vi "AB_Engine_Copy_Error_Files.vi"(8 "error in (no error)":errorcluster, 10 "preview only?":bool, 11 "Error destination path":path) -> (0 "error out":errorcluster, 3 "copied error files":path[](array[path]))   [LabVIEW 2020]
doc: "If \"Error destination path\" is empty, the computed RTE location is used."
uses:
  <resource>/Framework/Providers/Common/provcom_StringGlobals.vi
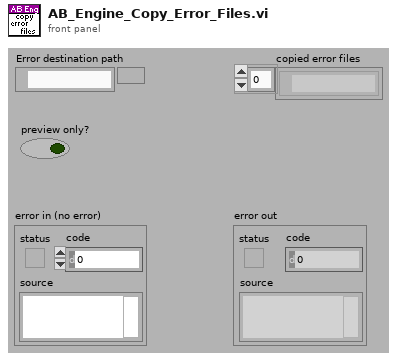
[diagram p1: front panel]
types:
  T1 = cluster{"base path":path, "relative path":path}[]
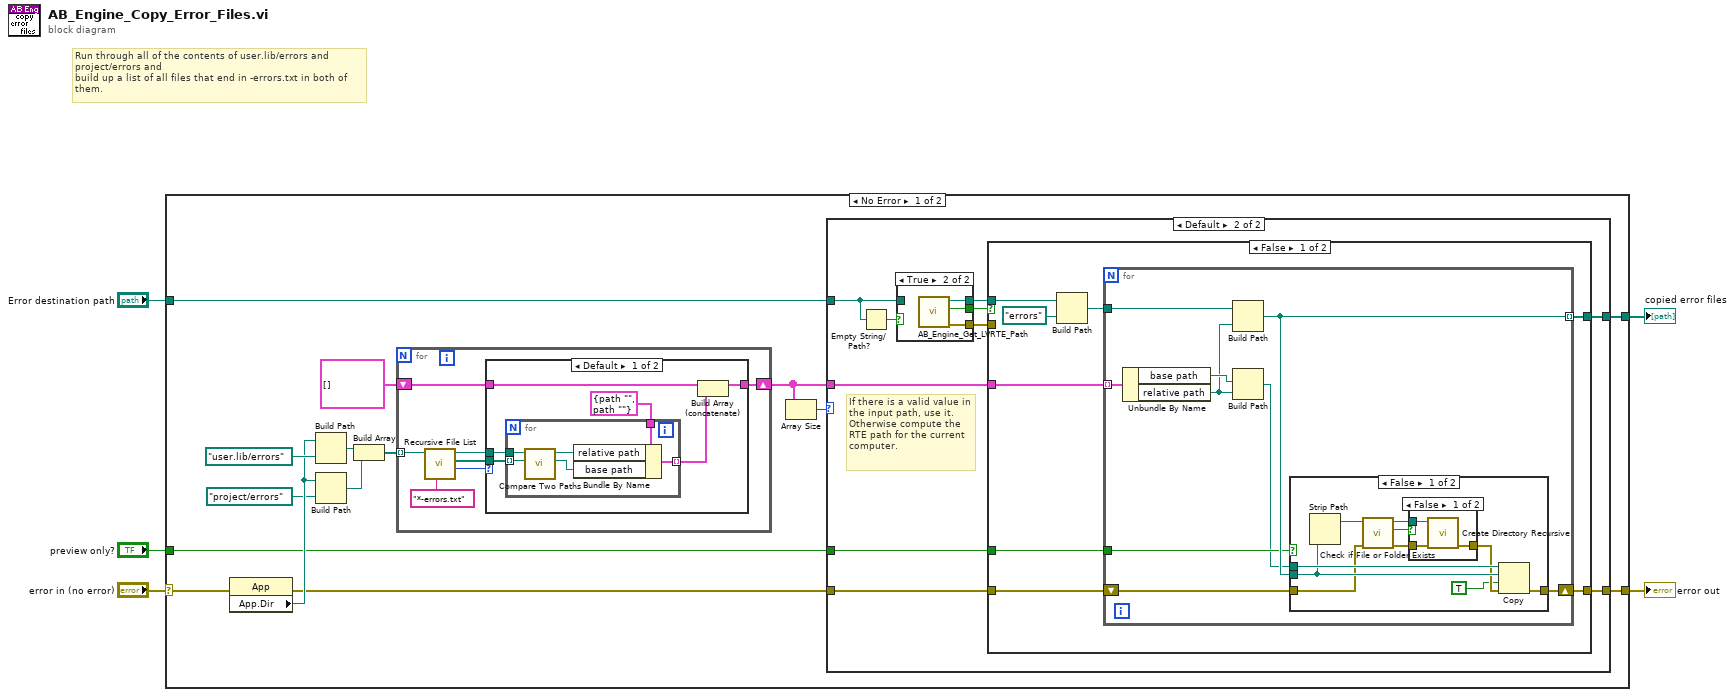
[diagram p0: block diagram]
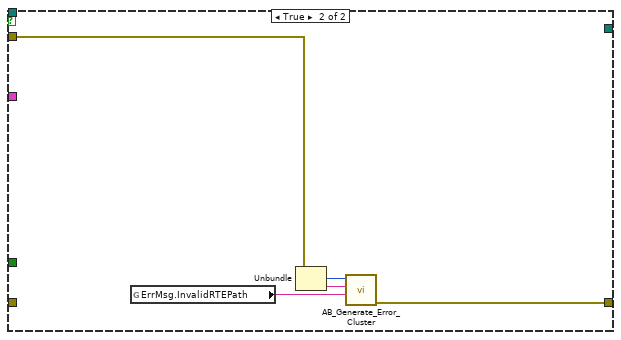
[diagram p5: hidden frame]
diagram:
  # "Run through all of the contents of user.lib/errors and project/errors and\nbuild up a list of all files that end in -errors.txt in both of them."
  n1 = case shown="No Error" "error in (no error)" {
    selector: "error in (no error)" -> [w19 w93]
    tunnel: [w20 w93] -> w4
    tunnel: "Error destination path" -> [w6 _]
    tunnel: [w11 _] -> w2
    tunnel: "preview only?" -> [w10 _]
    frame No Error {
      n2 = property class="App"(error in=w19) -> (error out=w9:errorcluster, "App.Dir"=w17:path)  [unwired: 1 in, 1 out]
      n3 = Build Path(base path=w17, name or relative path=path "user.lib/errors") -> (appended path=w15:path)
      n4 = Build Path(base path=w17, name or relative path=path "project/errors") -> (appended path=w14:path)
      n5 = Build Array(w15, w14) -> (w13:path[])
      n6 = for {
        shift-right: [w74] -> w8
        shift-left: T1 [] -> [w79]
        tunnel: w13 -> [w78] mode=indexing
        n7 = call <vilib>:"Recursive File List.vi"("pattern"="*-errors.txt" ("regular expression"), "Folder Path"=w78) -> ("Number of Files"=w76:i32, "All Files in Dir"=w75:path[], "dup Folder Path"=w73:path)  [unwired: 5 in, 2 out]
        n8 = case shown="Default" w76 {
          tunnel: [w85 w92] -> w74
          tunnel: w79 -> [w84 w92]
          tunnel: w75 -> [w83 _]
          tunnel: w73 -> [w82 _]
          frame Default {
            n9 = for {
              tunnel: w82 -> [w91]
              tunnel: w83 -> [w90] mode=indexing
              tunnel: [w87] -> w81 mode=indexing
              tunnel: cluster{"base path":path, "relative path":path} {"base path"=path "", "relative path"=path ""} -> [w86]
              n10 = call <vilib>:"Compare Two Paths.vi"("Path 2"=w90, "Path 1"=w91) -> ("Common Path"=w89:path, "Relative Path from 1 to 2"=w88:path)  [unwired: 6 in, 2 out]
              n11 = Bundle By Name(cluster=w86, "relative path"=w88, "base path"=w89) -> (w87:cluster{"base path":path, "relative path":path})
            }
            n12 = Build Array (concatenate)(w84, w81) -> (w85:T1)
          }
          frame 0 {
          }
        }
      }
      n13 = Array Size(array=w8) -> (size(s)=w7:i32)
      n14 = case shown="Default" w7 {
        tunnel: [w21 w31] -> w20
        tunnel: [_ w30] -> w11
        tunnel: w10 -> [_ w29]
        tunnel: w9 -> [w21 w28]
        tunnel: w6 -> [_ w24]
        tunnel: w8 -> [_ w27]
        frame 0 {
          # "If there are no files to copy, don't do anything."
        }
        frame Default {
          # "If there is a valid value in the input path, use it. Otherwise compute the RTE path for the current computer."
          n15 = Empty String/Path?(string/path=w24) -> (empty?=w26:bool)
          n16 = case shown="True" w26 {
            tunnel: w24 -> [w69 _]
            tunnel: [w69 w72] -> w25
            tunnel: [_ w71] -> w23
            tunnel: [_ w70] -> w22
            frame False {
            }
            frame True {
              n17 = call <vilib>:"AB_Engine_Get_LVRTE_Path.vi"() -> ("error out"=w70:errorcluster, "invalid RTE path?"=w71:bool, "Run-Time Engine Path"=w72:path)  [unwired: 9 in]
            }
          }
          n18 = case shown="False" w23 {
            tunnel: [w39 w68] -> w31
            tunnel: [w38 _] -> w30
            tunnel: w29 -> [w37 _]
            tunnel: w28 -> [w36 _]
            tunnel: w27 -> [w33 _]
            tunnel: w25 -> [w32 _]
            tunnel: w22 -> [_ w67]
            frame False {
              n19 = Build Path(base path=w32, name or relative path=path "errors") -> (appended path=w34:path)
              n20 = for {
                tunnel: w33 -> [w42] mode=indexing
                shift-right: [w48] -> w39
                shift-left: w36 -> [w47]
                tunnel: [w46] -> w38 mode=indexing
                tunnel: w37 -> [w45]
                tunnel: w34 -> [w44]
                n21 = Unbundle By Name(w42) -> ("base path"=w41:path, "relative path"=w40:path)
                n22 = Build Path(base path=w44, name or relative path=w40) -> (appended path=w46:path)
                n23 = Build Path(base path=w41, name or relative path=w40) -> (appended path=w43:path)
                n24 = case shown="False" w45 {
                  tunnel: w43 -> [w58 _]
                  tunnel: [w57 w63] -> w48
                  tunnel: w47 -> [w54 w63]
                  tunnel: w46 -> [w56 _]
                  frame False {
                    n25 = Strip Path(path=w56) -> (stripped path=w55:path)  [unwired: 1 out]
                    n26 = call <vilib>:"Check if File or Folder Exists.vi"("error in (no error)"=w54, "path"=w55) -> ("error out"=w52:errorcluster, "file or folder exists?"=w53:bool, "dup path"=w50:path)  [unwired: 7 in]
                    n27 = case shown="False" w53 {
                      tunnel: w52 -> [w61 w62]
                      tunnel: [w60 w62] -> w51
                      tunnel: w50 -> [w59 _]
                      frame False {
                        n28 = call <vilib>:"Create Directory Recursive.vi"("error in (no error)"=w61, "directory"=w59) -> ("error out"=w60:errorcluster)  [unwired: 3 in, 2 out]
                      }
                      frame True {
                      }
                    }
                    n29 = Copy(8:w51, 9:TRUE ("overwrite (F)"), 10:w56, 11:w58) -> (0:w57:errorcluster)  [unwired: 1 in, 2 out]
                  }
                  frame True {
                  }
                }
              }
            }
            frame True {
              n30 = global read "provcom_StringGlobals.vi" "ErrMsg.InvalidRTEPath"() -> (w64:string)
              n31 = Unbundle(w67) -> ("code"=w66:i32, "source"=w65:string)  [unwired: 1 out]
              n32 = call <vilib>:"AB_Generate_Error_Cluster.vi"("Additional Message"=w64, "source"=w65, "Code"=w66) -> ("error out"=w68:errorcluster)  [unwired: 1 in, 7 out]
            }
          }
        }
      }
    }
    frame Error {
    }
  }
  "error out" <- w4
  "copied error files" <- w2
